vi "Day 16-Binary String to Number.vi"(11 "Substring":string) -> (3 "Numeric":u64)   [LabVIEW 2021]
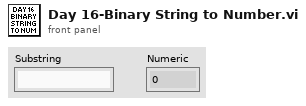
[diagram p1: front panel]
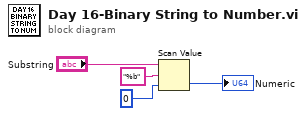
[diagram p0: block diagram]
diagram:
  n1 = Scan Value(string="Substring", format string="%b" ("string"), default (0 dbl)=u64 0) -> (value=→"Numeric":u64)  [unwired: 1 out]
